vi "SLSC_Command_Out.vi"(5 "Detect?":bool[](array[boolean]), 6 "SLSC Dynamic Commands":T1[](array[typedef]), 7 "Timeout?":bool, 8 "error in":errorcluster, 9 "Values":dbl[](array[numeric]), 10 "session in":refnum<k21>, 11 "SLSC Module Name":refnum<k21>) -> (0 "error out":errorcluster, 2 "session out":refnum<k21>, 3 "SLSC Module Name":refnum<k21>)   [LabVIEW 2020, in "SLSC-12201 DIO Engine.lvlib"]
uses:
  SLSC-12201 DIO Engine.lvlib
  Shared/SLSC Dynamic Channel.ctl
  Shared/SLSC Dynamic Channel Type.ctl
  <vilib>/SLSC/Execute Device Command.vi
  <vilib>/SLSC/Execute Phys Chan Command.vi
  <vilib>/SLSC/SLSC.lvlib
  <vilib>/NI VeriStand/Custom Device Tools/Custom Device Utility Library/Custom Device Utility Library.lvlib
  Shared/SLSC-12201 DIO Shared.lvlib
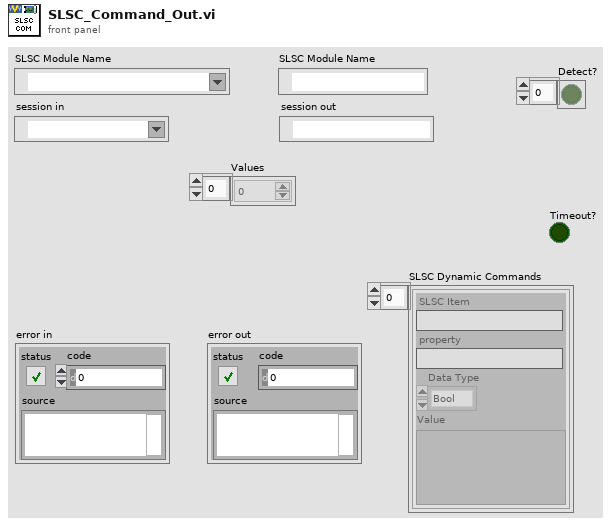
[diagram p1: front panel]
types:
  T1 = typedef "SLSC-12201 DIO Shared.lvlib/SLSC Dynamic Channel.ctl" = cluster{"SLSC Item":string, "property":string, "Data Type":T2, "Value":variant}
  T2 = typedef "SLSC-12201 DIO Shared.lvlib/SLSC Dynamic Channel Type.ctl" = enum16{"Bool", "Double", "I32", "I64", "String", "U32", "U64", "EnumI32"}
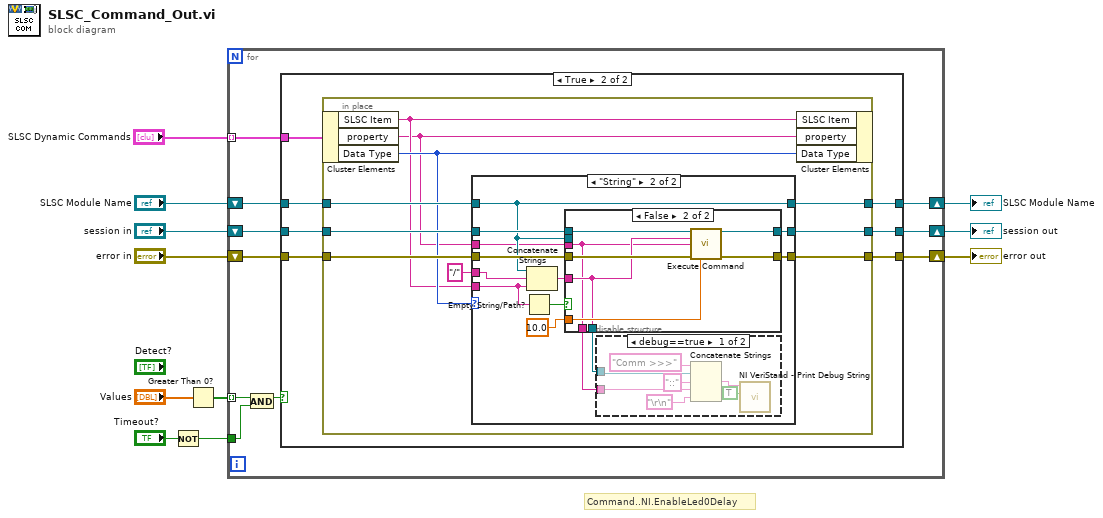
[diagram p0: block diagram]
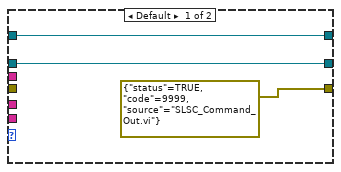
[diagram p3: hidden frame]
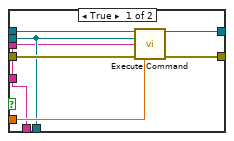
[diagram p5: hidden frame]
diagram:
  # "Command..NI.EnableLed0Delay"
  n1 = Not(x="Timeout?") -> (.not. x?=w1:bool)
  n2 = Greater Than 0?(x="Values") -> (x > 0?=w3:bool[])
  n3 = for {
    tunnel: "SLSC Dynamic Commands" -> [w21] mode=indexing
    shift-right: [w19] -> w6
    shift-left: "session in" -> [w20]
    shift-right: [w17] -> w8
    shift-left: "SLSC Module Name" -> [w18]
    shift-right: [w15] -> w5
    shift-left: "error in" -> [w16]
    tunnel: w3 -> [w14] mode=indexing
    tunnel: w1 -> [w12]
    n4 = And(x=w14, y=w12) -> (x .and. y?=w13:bool)
    n5 = case shown="True" w13 {
      tunnel: w21 -> [_ w25]
      tunnel: w20 -> [w23 w31]
      tunnel: [w23 w30] -> w19
      tunnel: w18 -> [w24 w29]
      tunnel: [w24 w28] -> w17
      tunnel: w16 -> [w22 w27]
      tunnel: [w22 w26] -> w15
      frame False {
      }
      frame True {
        n6 = in-place {
          in-place-border: w31 -> [w41]
          in-place-border: [w40] -> w30
          in-place-border: w29 -> [w39]
          in-place-border: [w38] -> w28
          in-place-border: w27 -> [w37]
          in-place-border: [w36] -> w26
          n7 = in-place-cluster #1(w25) -> ("SLSC Item"=w33:string, "property"=w32:string, "Data Type"=w34:T2)
          n8 = case shown="\"String\"" w34 {
            tunnel: w41 -> [w43 w53]
            tunnel: [w43 w56] -> w40
            tunnel: w33 -> [_ w47]
            tunnel: w39 -> [w44 w50]
            tunnel: [w44 w50] -> w38
            tunnel: w37 -> [_ w52]
            tunnel: [errorcluster {"status"=TRUE, "code"=9999, "source"="SLSC_Command_Out.vi"} ("error out") w55] -> w36
            tunnel: "/" -> [_ w57]
            tunnel: w32 -> [_ w49]
            frame Default {
            }
            frame "String" {
              n9 = Empty String/Path?(string/path=w47) -> (empty?=w51:bool)
              n10 = Concatenate Strings(w50, w57, w47) -> (w48:string)
              n11 = case shown="False" w51 {
                tunnel: w53 -> [w71 w78]
                tunnel: [w70 w77] -> w56
                tunnel: [w69 w76] -> w55
                tunnel: 10.0 ("timeout (10 sec)") -> [w68 w75]
                tunnel: w52 -> [w67 w74]
                tunnel: w49 -> [w65 w72]
                tunnel: w48 -> [_ w73]
                tunnel: w50 -> [w66 _]
                tunnel: [w66 w73] -> w46
                tunnel: [w65 w72] -> w45
                frame True {
                  n12 = call-poly <vilib>:"Execute Command.vi"("session in"=w71, "devices"=w66, "command"=w65, "error in (no error)"=w67, "timeout (10 sec)"=w68) -> ("session out"=w70:refnum<k21>, "error out"=w69:errorcluster)  [unwired: 9 in]
                }
                frame False {
                  n13 = call-poly <vilib>:"Execute Command.vi"("session in"=w78, "physical channels"=w73, "command"=w72, "error in (no error)"=w74, "timeout (10 sec)"=w75) -> ("session out"=w77:refnum<k21>, "error out"=w76:errorcluster)  [unwired: 9 in]
                }
              }
              n14 = disable-structure shown="debug==true" {
                disable-tunnel: w45 -> [w59 _]
                disable-tunnel: w46 -> [w62 _]
                frame condition #0 {
                  n15 = Concatenate Strings("Comm >>>" ("string"), w62, "::" ("string"), w59, "\r\n") -> (w63:string)
                  n16 = call <vilib>:"NI VeriStand - Print Debug String.vi"("Add to log file? (F)"=TRUE ("Add to log file? (T)"), "Message"=w63) -> ()  [unwired: 9 in, 1 out]
                }
                frame condition #1 (active) {
                }
              }
            }
          }
          n17 = in-place-cluster #1("SLSC Item"=w33, "property"=w32, "Data Type"=w34) -> ()  [unwired: 1 out]
        }
      }
    }
  }
  "error out" <- w5
  "session out" <- w6
  "SLSC Module Name" <- w8
